vi "Calculate Overall Status.vi"(10 "Status Calculation":T1, 11 "Status's":T2[](array[typedef])) -> (2 "Overall Status":T2)   [LabVIEW 2021, in "BT.lvlib" / "bt_Parallel.lvclass"]
uses:
  bt_Parallel.lvclass
  abs_Node/Status.ctl
  Status Calculation.ctl
  abs_Node/bt_Node.lvclass
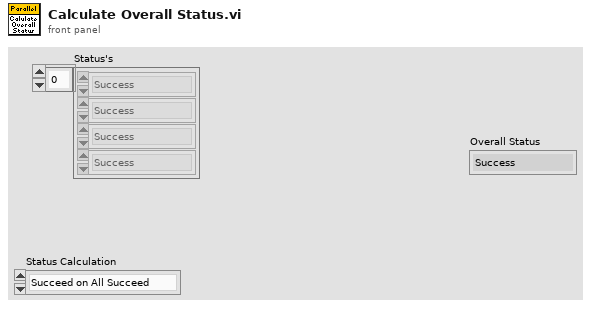
[diagram p1: front panel]
types:
  T1 = typedef "BT.lvlib/bt_Parallel.lvclass/Status Calculation.ctl" = enum16{"Succeed on All Succeed", "Failure on All Failure", "Succeed on Any Succeed", "Failure on Any Failure"}
  T2 = typedef "BT.lvlib/bt_Node.lvclass/Status.ctl" = enum16{"Success", "Failure", "Running"}
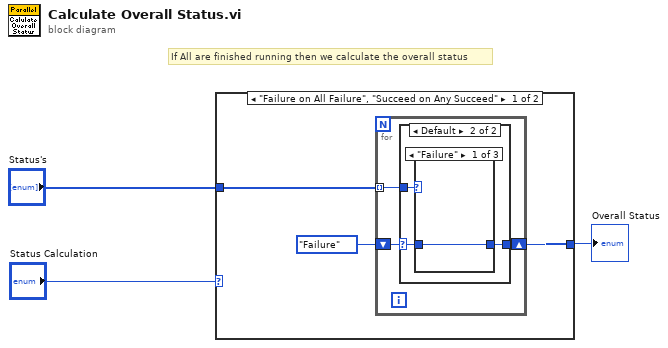
[diagram p0: block diagram]
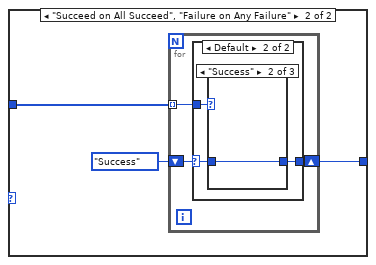
[diagram p5: hidden frame]
diagram:
  # "If All are finished running then we calculate the overall status"
  n1 = case shown="\"Failure on All Failure\", \"Succeed on Any Succeed\"" "Status Calculation" {
    tunnel: "Status's" -> [w6 w19]
    tunnel: [w5 w18] -> w3
    frame "Failure on All Failure", "Succeed on Any Succeed" {
      n2 = for {
        tunnel: w6 -> [w9] mode=indexing
        shift-right: [w8] -> w5
        shift-left: Status."Failure" ("Status") -> [w7]
        n3 = case shown="Default" w7 {
          selector: w7 -> [w10 w11]
          tunnel: w9 -> [_ w13]
          tunnel: [w10 w12] -> w8
          frame "Running" {
          }
          frame Default {
            n4 = case shown="\"Failure\"" w13 {
              selector: w13 -> [_ w15 w16]
              tunnel: [w14 w15 w16] -> w12
              tunnel: w11 -> [w14 _ _]
              frame "Failure" {
              }
              frame "Success" {
              }
              frame "Running" {
              }
            }
          }
        }
      }
    }
    frame "Succeed on All Succeed", "Failure on Any Failure" {
      n5 = for {
        tunnel: w19 -> [w22] mode=indexing
        shift-right: [w21] -> w18
        shift-left: Status."Success" ("Status") -> [w20]
        n6 = case shown="Default" w20 {
          selector: w20 -> [w23 w24]
          tunnel: w22 -> [_ w26]
          tunnel: [w23 w25] -> w21
          frame "Running" {
          }
          frame Default {
            n7 = case shown="\"Success\"" w26 {
              selector: w26 -> [w27 _ w29]
              tunnel: [w27 w28 w29] -> w25
              tunnel: w24 -> [_ w28 _]
              frame "Failure" {
              }
              frame "Success" {
              }
              frame "Running" {
              }
            }
          }
        }
      }
    }
  }
  "Overall Status" <- w3
